vi "Upd State.vi"(8 "error in (no error)":errorcluster, 10 "Upd State":bool, 11 "TCP 380 in":refnum<class "TCP 380.lvclass">) -> (0 "error out":errorcluster, 3 "TCP 380 out":refnum<class "TCP 380.lvclass">)   [LabVIEW 2021, in "TCP 380.lvclass"]
uses:
  TCP 380.lvclass
  TCP 380.lvclass/TCP 380.ctl
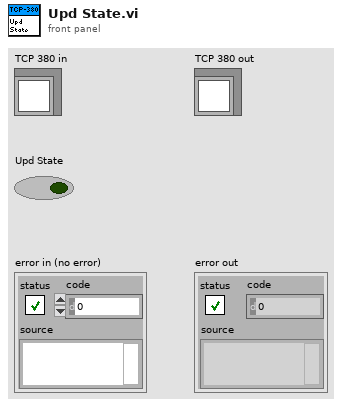
[diagram p1: front panel]
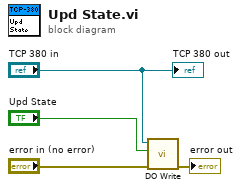
[diagram p0: block diagram]
diagram:
  n1 = call "DO Write.vi"("error in (no error)"="error in (no error)", "Digital Output"="Upd State", "TCP 380 in"="TCP 380 in") -> ("error out"=→"error out":errorcluster)  [unwired: 8 in]
  "TCP 380 out" <- "TCP 380 in"
